vi "rs3 Advanced set Rau Threshold3.vi"(8 "error in (no error)":errorcluster, 10 "ST Rau Threshold":T1, 11 "device in":u64) -> (0 "error out":errorcluster, 1 "error":u64, 3 "Dev out":u64)   [LabVIEW 2019, in "libRealSense3.lvlib"]
doc: "This sets some register that affect the depth calculations"
uses:
  libRealSense3.lvlib
  realsense2.dll
panel:
  # "RS3 Adv. Set RAU Threshold2"
  # "(C) 2017 Intel Corp.,  AGJ"
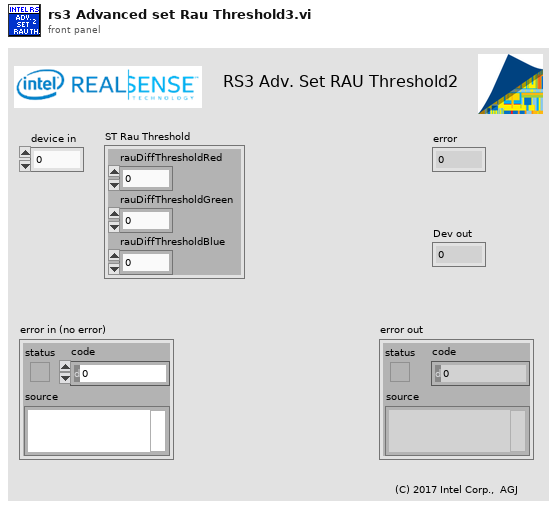
[diagram p1: front panel]
types:
  T1 = cluster{"rauDiffThresholdRed":u32, "rauDiffThresholdGreen":u32, "rauDiffThresholdBlue":u32}
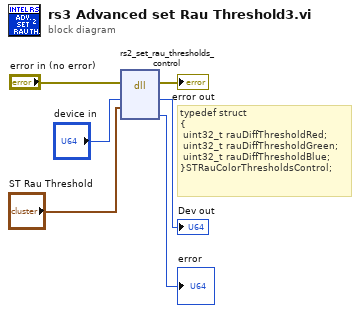
[diagram p0: block diagram]
diagram:
  # "typedef struct\n{\n\tuint32_t rauDiffThresholdRed;\n\tuint32_t rauDiffThresholdGreen;\n\tuint32_t rauDiffThresholdBlue;\n}STRauColorThresholdsControl;"
  n1 = dll-call lib="C:/Users/morte/Documents/gitmoro/treadmill/RealSense for Labview ver. 2.33/realsense2.dll" fn="rs2_set_rau_thresholds_control"(error in="error in (no error)", "device"="device in", "ST Rau Threshold"="ST Rau Threshold") -> (error out=→"error out":errorcluster, "device"=→"Dev out":u64, "error"=→"error":u64)  [unwired: 5 in, 1 out]
